vi "sub_resample_and_demodulate_Temp.vi"(4 "packet_array":cdb[][](array[numeric]), 5 "Rx IQ Sampling Rate [s/sec]":dbl, 6 "error in (no error)":errorcluster, 9 "PSK Init Parameters":T2) -> (0 "error out":errorcluster, 1 "recovered complex waveform":T1[](array[typedef]) {"Y" format="%.3f"; "dt" format="%^.2e"; "t0" format="%.4f"}, 2 "output bit stream":i8[][](array[numeric]), 3 "Sync Found":bool)   [LabVIEW 2013]
uses:
  <vilib>/addons/Modulation/Analog/controls/Complex Data Waveform.ctl
  <vilib>/addons/Modulation/niAMT.lvlib
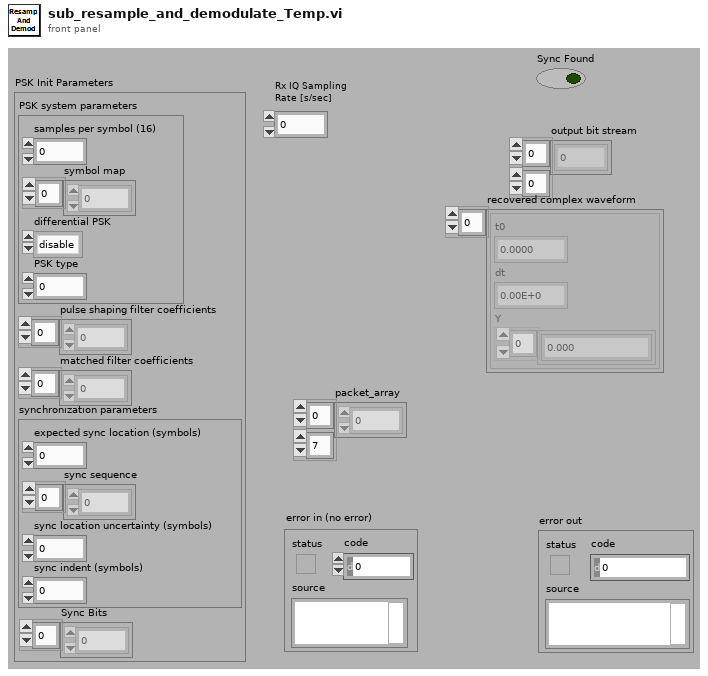
[diagram p1: front panel]
types:
  T1 = typedef "niAMT.lvlib/Complex Data Waveform.ctl" = cluster{"t0":dbl, "dt":dbl, "Y":cdb[]}
  T2 = cluster{"PSK system parameters":cluster{"samples per symbol (16)":i32, "symbol map":cdb[], "differential PSK":enum16{"disable", "enable"}, "PSK type":u16}, "pulse shaping filter coefficients":dbl[], "matched filter coefficients":dbl[], "synchronization parameters":cluster{"expected sync location (symbols)":i32, "sync sequence":cdb[], "sync location uncertainty (symbols)":i32, "sync indent (symbols)":i32}, "Sync Bits":i8[]}
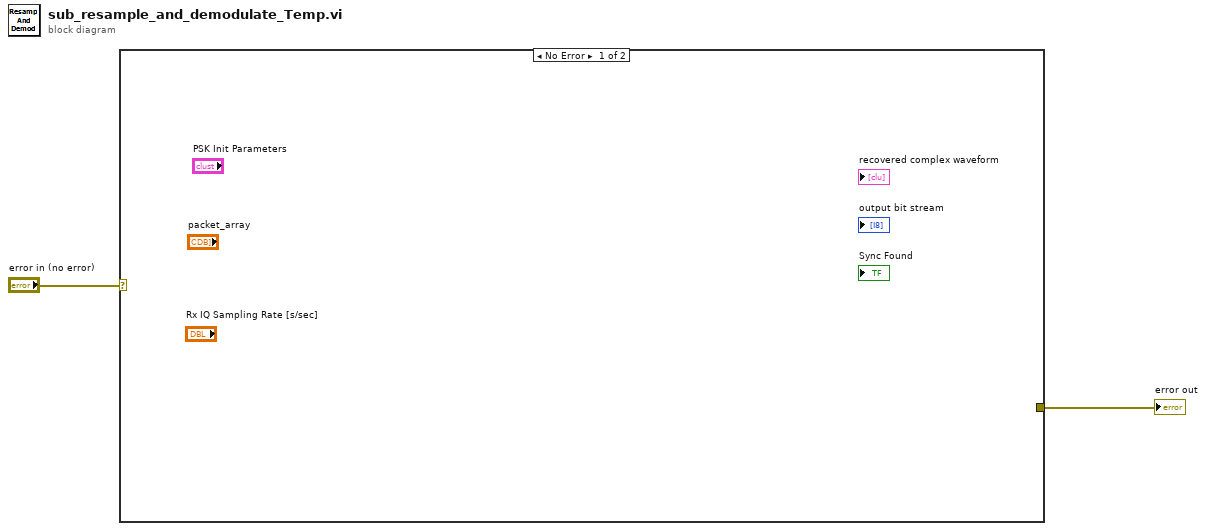
[diagram p0: block diagram]
diagram:
  n1 = case shown="No Error" "error in (no error)" {
    selector: "error in (no error)" -> [_ w3]
    tunnel: [_ w3] -> w2
    frame No Error {
    }
    frame Error {
    }
  }
  "error out" <- w2
